vi "createLogFile (SubVI).vi"(4 "trial #":i32, 5 "1st Handle Left?":bool, 6 "directory Path":path, 7 "Subject ID":T1, 8 "unit":T2, 9 "count in unit":i32, 10 "unit #":i32) -> (3 "file path out":path)   [LabVIEW 2011]
uses:
  ctlProtocolUnit.ctl
  ctlProtocolSubID.ctl
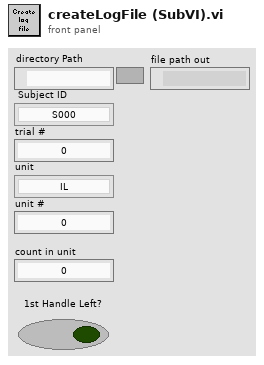
[diagram p1: front panel]
types:
  T1 = typedef "ctlProtocolSubID.ctl" = enum16{"S000", "S001", "S002", "S003", "S004", "S005", "S006", "S007", "S008", "S009", "S010", "S011", "S012", "S013", "S014", "S015", "S016", "S017", "S018", "S019", "S020", "S021", "S022", "S023", "S024", "S025", "S026", "S027", "S028", "S029", "S030"}
  T2 = typedef "ctlProtocolUnit.ctl" = enum16{"IL", "TR", "PT"}
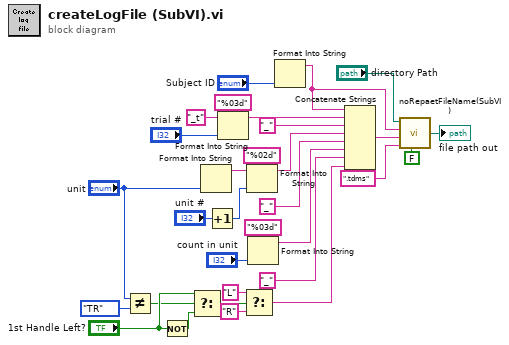
[diagram p0: block diagram]
diagram:
  n1 = Not Equal?(x="unit", y=ctlProtocolUnit."TR" ("Protocol.unit")) -> (x != y?=w27:bool)
  n2 = Not(x="1st Handle Left?") -> (.not. x?=w26:bool)
  n3 = Select(t="1st Handle Left?", s=w27, f=w26) -> (s? t:f=w23:bool)
  n4 = Format Into String("unit") -> (resulting string=w15:string)  [unwired: 3 in, 1 out]
  n5 = Increment(x="unit #") -> (x+1=w18:i32)
  n6 = Format Into String(format string="%03d", initial string="_t", "trial #") -> (resulting string=w16:string)  [unwired: 1 in, 1 out]
  n7 = Select(t="L", s=w23, f="R") -> (s? t:f=w11:string)
  n8 = Format Into String(format string="%02d", initial string=w15, w18) -> (resulting string=w14:string)  [unwired: 1 in, 1 out]
  n9 = Format Into String(format string="%03d", "count in unit") -> (resulting string=w13:string)  [unwired: 2 in, 1 out]
  n10 = Format Into String("Subject ID") -> (resulting string=w10:string)  [unwired: 3 in, 1 out]
  n11 = Concatenate Strings(w10, w16, "_" ("string"), w14, "_" ("string"), w13, "_" ("string"), w11) -> (w8:string)
  n12 = call "noRepaetFileName(SubVI).vi"("prompt overwrite?"=FALSE, "ext"=".tdms", "file name"=w8, "subID"=w10, "directory Path"="directory Path") -> ("file path out"=→"file path out":path)  [unwired: 1 in]
